vi "add and map fixed channel mapping.vi"(7 "action instance":string, 8 "error in":errorcluster, 10 "fixed channel":refnum<class "TBM channel.lvclass">, 11 "engine configuration in":refnum<class "base TBM sequencer configuration.lvclass">) -> (0 "error out":errorcluster, 3 "engine configuration out":refnum<class "base TBM sequencer configuration.lvclass">)   [LabVIEW 2014, in "base TBM sequencer configuration.lvclass"]
uses:
  base TBM sequencer configuration.lvclass
  <vilib>/NI/Tag Bus Module Framework/channel/TBM channel.lvclass
  <vilib>/NI/Tag Bus/tag/tag descriptor.lvclass/tag descriptor.ctl
  <vilib>/NI/Tag Bus/tag/read tag name.vi
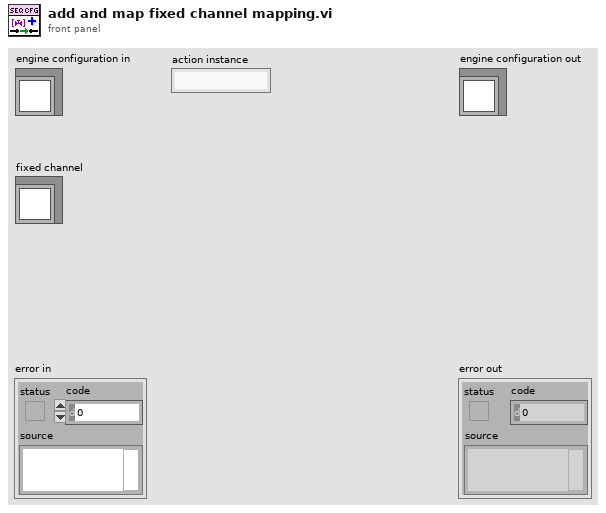
[diagram p1: front panel]
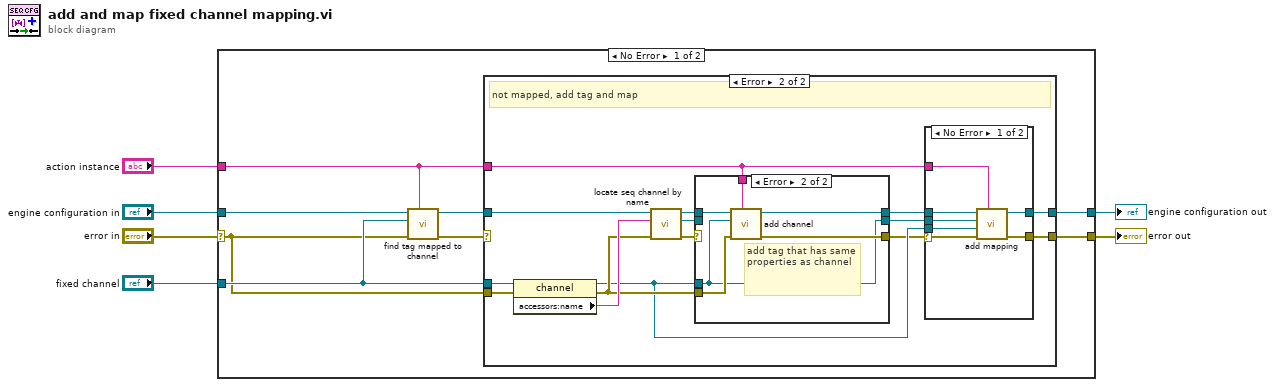
[diagram p0: block diagram]
diagram:
  n1 = case shown="No Error" "error in" {
    selector: "error in" -> [w7 w51]
    tunnel: [w9 w51] -> w5
    tunnel: [w10 w50] -> w3
    tunnel: "engine configuration in" -> [w14 w50]
    tunnel: "fixed channel" -> [w8 _]
    tunnel: "action instance" -> [w13 _]
    frame No Error {
      n2 = call "find tag mapped to channel.vi"("owner"=w13, "error in"=w7, "action channel"=w8, "engine configuration in"=w14) -> ("error out"=w12:errorcluster, "engine configuration out"=w11:refnum<class "base TBM sequencer configuration.lvclass">)  [unwired: 5 in, 1 out]
      n3 = case shown="Error" w12 {
        selector: w12 -> [w15 _]
        tunnel: w13 -> [_ w19]
        tunnel: w8 -> [_ w31]
        tunnel: w7 -> [_ w30]
        tunnel: w11 -> [w16 w28]
        tunnel: [w16 w22] -> w10
        tunnel: [w15 w21] -> w9
        frame No Error {
          # "Already mapped, do nothing"
        }
        frame Error {
          # "not mapped, add tag and map"
          n4 = property class="channel"(reference=w31, error in=w30) -> (reference out=w18:refnum<class "TBM channel.lvclass">, error out=w26:errorcluster, "accessors:name"=w29:string)
          n5 = call "locate seq channel by name.vi"("error in"=w26, "channel name"=w29, "engine configuration in"=w28) -> ("error out"=w27:errorcluster, "channel descriptor"=w25:refnum<class "TBM channel.lvclass">, "engine configuration out"=w24:refnum<class "base TBM sequencer configuration.lvclass">)  [unwired: 6 in]
          n6 = case shown="Error" w27 {
            selector: w27 -> [w41 _]
            tunnel: w26 -> [_ w47]
            tunnel: w19 -> [_ w48]
            tunnel: [w43 w44] -> w20
            tunnel: w25 -> [w43 _]
            tunnel: w24 -> [w42 w49]
            tunnel: [w42 w46] -> w23
            tunnel: [w41 w45] -> w17
            tunnel: w18 -> [_ w44]
            frame No Error {
              # "tag exists, map"
            }
            frame Error {
              # "add tag that has same properties as channel"
              n7 = call "add channel.vi"("owner ID"=w48, "error in"=w47, "channel descriptor"=w44, "engine configuration in"=w49) -> ("error out"=w45:errorcluster, "engine configuration out"=w46:refnum<class "base TBM sequencer configuration.lvclass">)  [unwired: 6 in]
            }
          }
          n8 = case shown="No Error" w17 {
            selector: w17 -> [w33 w39]
            tunnel: w23 -> [w38 w40]
            tunnel: [w37 w40] -> w22
            tunnel: [w36 w39] -> w21
            tunnel: w20 -> [w32 _]
            tunnel: w19 -> [w35 _]
            tunnel: w18 -> [w34 _]
            frame No Error {
              n9 = call "add mapping.vi"("owner ID"=w35, "error in"=w33, "action channel"=w34, "seq channel"=w32, "engine configuration"=w38) -> ("error out"=w36:errorcluster, "engine configuration out"=w37:refnum<class "base TBM sequencer configuration.lvclass">)  [unwired: 5 in]
            }
            frame Error {
              # "tag add failed"
            }
          }
        }
      }
    }
    frame Error {
    }
  }
  "error out" <- w5
  "engine configuration out" <- w3
